vi "ge_ChassisTree.vi"(6 "Child Position":i32, 7 "ge_TreeCmnd":T1, 8 "error in":errorcluster, 9 "Module Name":string, 10 "Chassis Name":string, 11 "Hardware":refnum<vi>) -> (0 "error out":errorcluster)   [LabVIEW 2012]
uses:
  Custom Ctrls/ge_ChassisTree.ctl
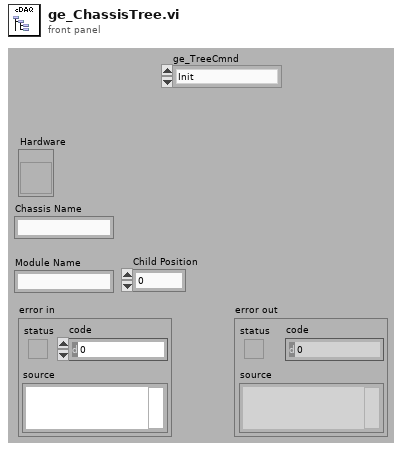
[diagram p1: front panel]
types:
  T1 = typedef "ge_ChassisTree.ctl" = enum16{"Init", "Add Chassis", "Add Mod", "Close"}
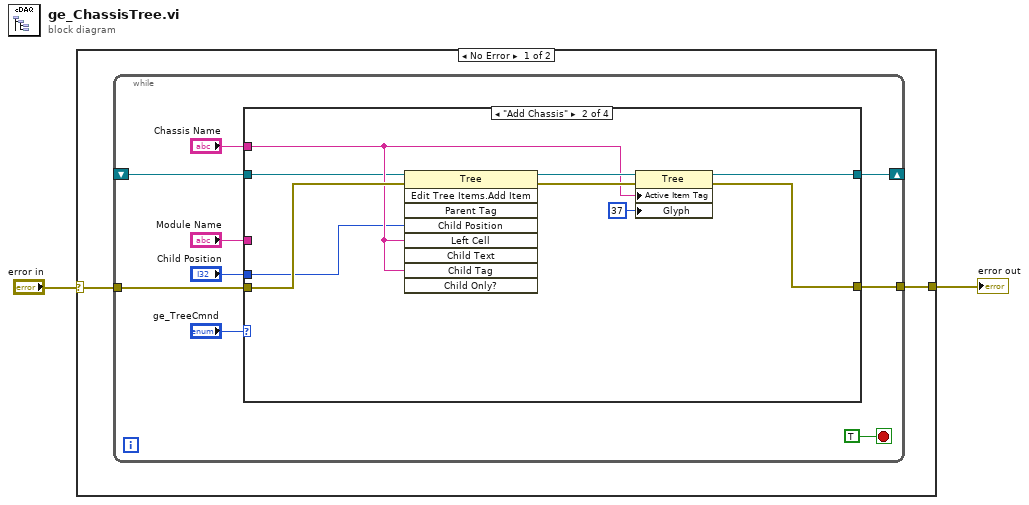
[diagram p0: block diagram]
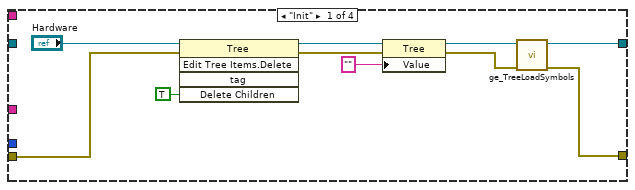
[diagram p2: hidden frame]
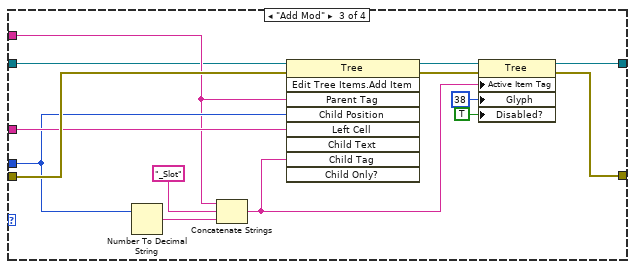
[diagram p3: hidden frame]
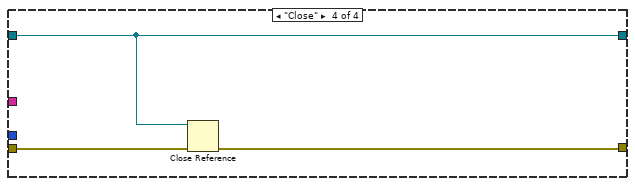
[diagram p4: hidden frame]
diagram:
  n1 = case shown="No Error" "error in" {
    selector: "error in" -> [w3 w50]
    tunnel: [w4 w50] -> w2
    frame No Error {
      n2 = while {
        tunnel: w3 -> [w9]
        tunnel: [w8] -> w4
        shift-right: [w13] -> _
        shift-left: _ -> [w5]
        stop <- TRUE stop-if-true
        n3 = case shown="\"Add Chassis\"" "ge_TreeCmnd" {
          tunnel: [w21 w29 w43 w47] -> w13
          tunnel: "Chassis Name" -> [_ w26 w34 _]
          tunnel: "Module Name" -> [_ _ w40 _]
          tunnel: w9 -> [w22 w32 w46 w49]
          tunnel: [w20 w28 w42 w48] -> w8
          tunnel: "Child Position" -> [_ w25 w39 _]
          tunnel: w5 -> [_ w24 w33 w47]
          frame "Init" {
            n4 = invoke on="Invoke Node" class="Tree" method="Edit Tree Items.Delete"(reference="Hardware", error in=w22, "Delete Children"=TRUE ("Delete Children?")) -> (reference out=w18:refnum<vi>, error out=w17:errorcluster)  [unwired: 2 in, 3 out]
            n5 = property class="Tree"(reference=w18, error in=w17, "Value"="") -> (reference out=w16:refnum<vi>, error out=w15:errorcluster)
            n6 = call "ge_TreeLoadSymbols.vi"("error in (no error)"=w15, "tree refnum"=w16) -> ("error out"=w20:errorcluster, "dup tree refnum"=w21:refnum<vi>)  [unwired: 6 in]
          }
          frame "Add Chassis" {
            n7 = invoke on="Invoke Node" class="Tree" method="Edit Tree Items.Add Item"(reference=w24, error in=w32, "Child Position"=w25, "Left Cell"=w26, "Child Tag"=w26) -> (reference out=w30:refnum<vi>, error out=w27:errorcluster)  [unwired: 4 in, 7 out]
            n8 = property class="Tree"(reference=w30, error in=w27, "Active Item Tag"=w26, "Glyph"=37 ("Active Item:Symbol Index")) -> (reference out=w29:refnum<vi>, error out=w28:errorcluster)
          }
          frame "Add Mod" {
            n9 = Number To Decimal String(number=w39) -> (decimal integer string=w38:string)  [unwired: 1 in]
            n10 = Concatenate Strings(w34, "_Slot" ("string"), w38) -> (w36:string)
            n11 = invoke on="Invoke Node" class="Tree" method="Edit Tree Items.Add Item"(reference=w33, error in=w46, "Parent Tag"=w34, "Child Position"=w39, "Left Cell"=w40, "Child Tag"=w36) -> (reference out=w45:refnum<vi>, error out=w44:errorcluster)  [unwired: 3 in, 7 out]
            n12 = property class="Tree"(reference=w45, error in=w44, "Active Item Tag"=w36, "Glyph"=38 ("Active Item:Symbol Index"), "Disabled?"=TRUE ("Active Item:Disabled?")) -> (reference out=w43:refnum<vi>, error out=w42:errorcluster)
          }
          frame "Close" {
            n13 = Close Reference(reference=w47, error in (no error)=w49) -> (error out=w48:errorcluster)
          }
        }
      }
    }
    frame Error {
    }
  }
  "error out" <- w2
